vi "Heartbeat pulse.vi"(4 "error in":errorcluster, 6 "Node ID":u8, 7 "CANopen in":refnum<class "CANopen.lvclass">) -> (0 "error out":errorcluster, 3 "CANopen out":refnum<class "CANopen.lvclass">)   [LabVIEW 2026, in "canopen_.lvlib" / "CANopen.lvclass"]
doc: "Decrements the watchdog of a specific heartbeat entry or of all the entries if \"Node ID\" is not specified. A negative \"Value\" in the entry indicates a watchdog alarm. Watchdog alarms are usually returned to the application by \"CAN refresh\"."
uses:
  CANopen.lvclass
  CANopen.lvclass/CANopen.ctl
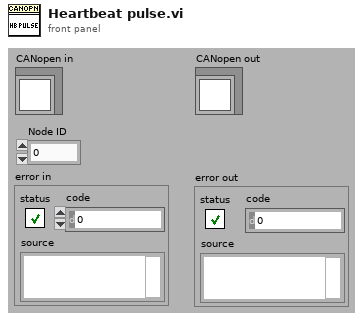
[diagram p1: front panel]
types:
  T1 = cluster{"Node ID":u8, "Period":u16, "Timeout":u16, "Last Beat":timestamp}[]
  T2 = cluster{"Node ID":u8, "Period":u16, "Timeout":u16, "Last Beat":timestamp}
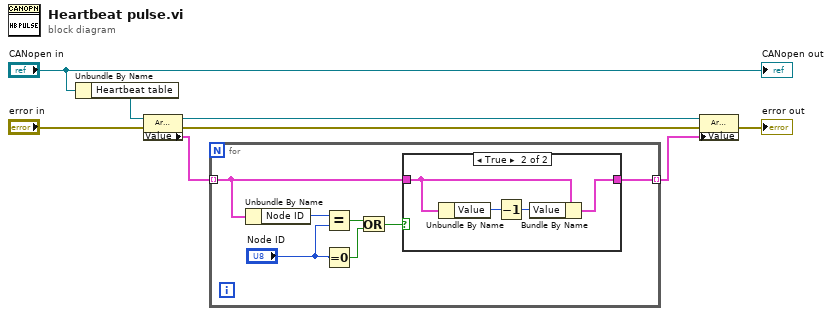
[diagram p0: block diagram]
diagram:
  n1 = Unbundle By Name("CANopen in") -> ("Heartbeat table"=w8:refnum<vi>)
  n2 = property class="Arr (strict)"(reference=w8, error in="error in") -> (reference out=w5:refnum<vi>, error out=w3:errorcluster, "Value"=w6:T1)
  n3 = for {
    tunnel: w6 -> [w11] mode=indexing
    tunnel: [w10] -> w4 mode=indexing
    n4 = Unbundle By Name(w11) -> ("Node ID"=w15:u8)
    n5 = Equal?(x=w15, y="Node ID") -> (x = y?=w13:bool)
    n6 = Equal To 0?(x="Node ID") -> (x = 0?=w12:bool)
    n7 = Or(x=w13, y=w12) -> (x .or. y?=w9:bool)
    n8 = case shown="True" w9 {
      tunnel: w11 -> [w16 w20]
      tunnel: [w16 w19] -> w10
      frame False {
      }
      frame True {
        n9 = Unbundle By Name(w20) -> ("Value"=w17:i16)
        n10 = Decrement(x=w17) -> (x-1=w18:i16)
        n11 = Bundle By Name(cluster=w20, "Value"=w18) -> (w19:T2)
      }
    }
  }
  n12 = property class="Arr (strict)"(reference=w5, error in=w3, "Value"=w4) -> (error out=→"error out":errorcluster)  [unwired: 1 out]
  "CANopen out" <- "CANopen in"
